vi "Min si Max Lab 2.vi"() -> ()   [LabVIEW 2023]
panel:
  out "Boolean":bool
  in  "Limitare":bool
  in  "MAX":dbl(slide) scale=0.0..10.0
  in  "MIN":dbl(slide) scale=0.0..10.0
  out "Tank":dbl(slide) scale=0.0..10.0
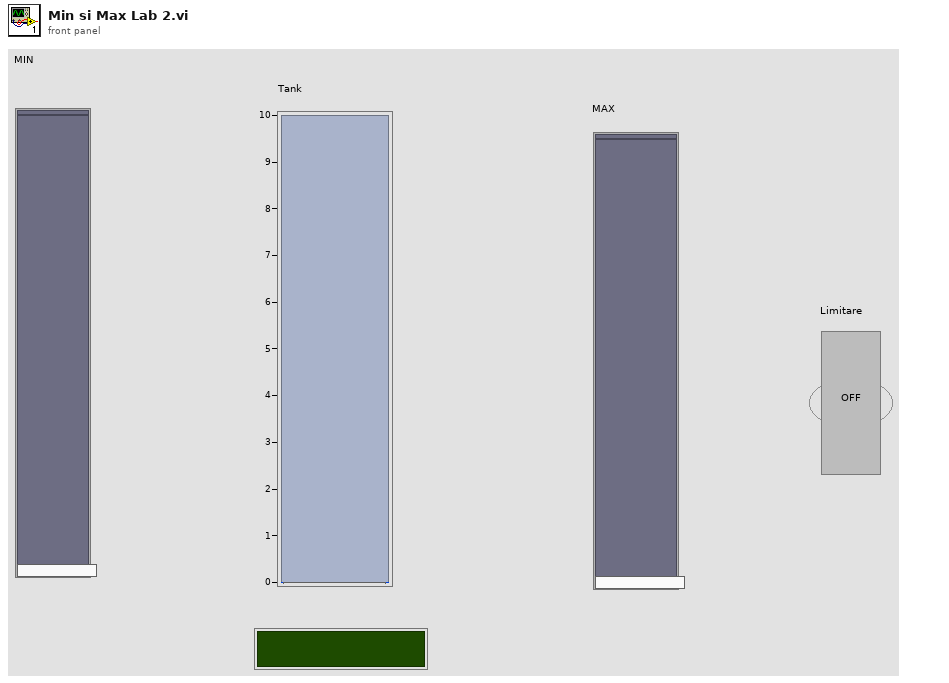
[diagram p1: front panel]
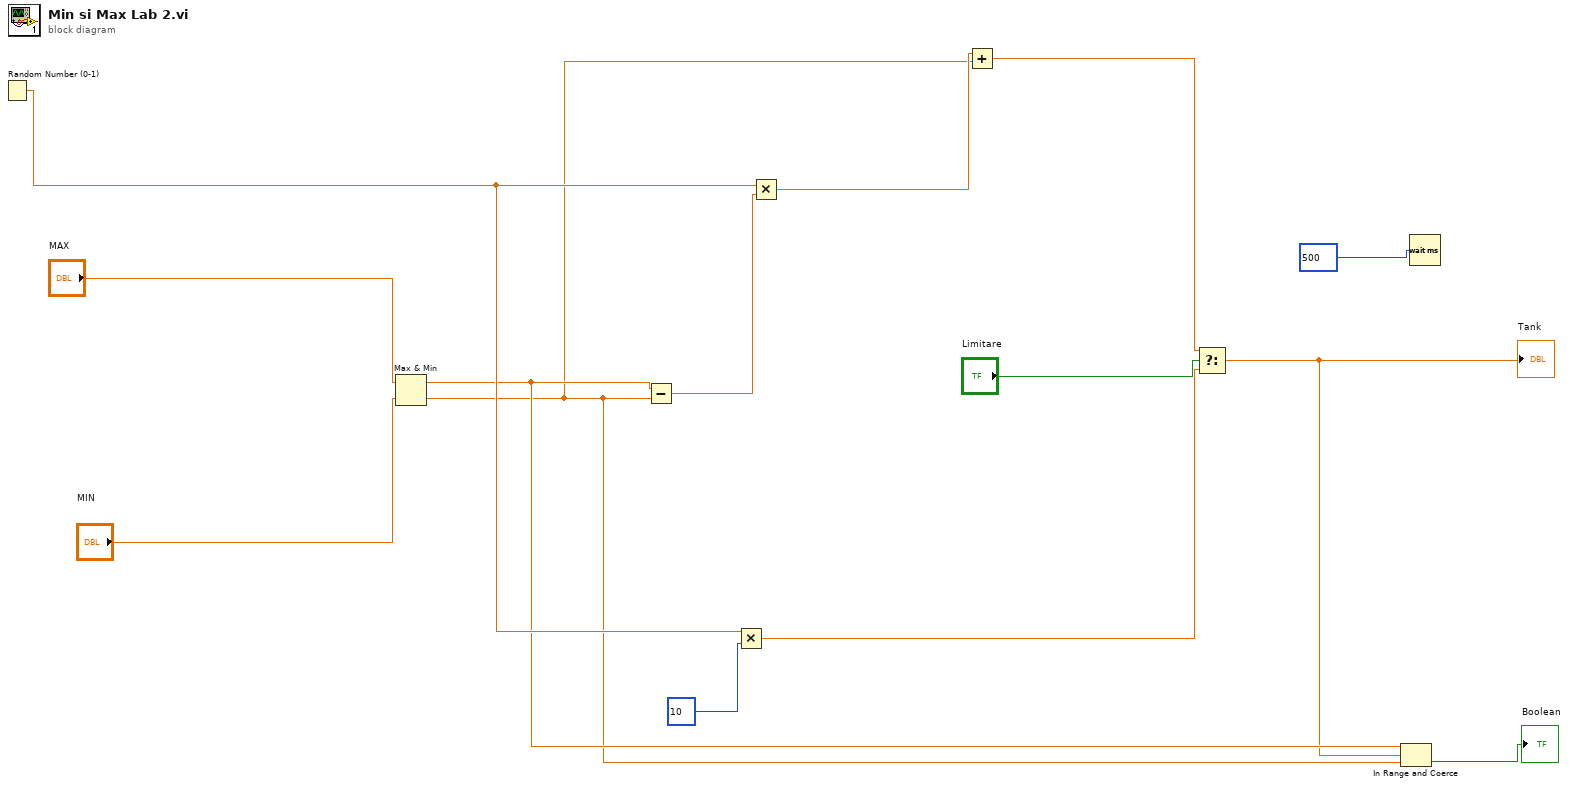
[diagram p0: block diagram]
diagram:
  n1 = Random Number (0-1)() -> (number: 0 to 1=w10:dbl)
  n2 = Max & Min(x="MAX", y="MIN") -> (max(x,y)=w5:dbl, min(x,y)=w3:dbl)
  n3 = Subtract(x=w5, y=w3) -> (x-y=w12:dbl)
  n4 = Multiply(x=w10, y=10) -> (x*y=w6:dbl)
  n5 = Multiply(x=w10, y=w12) -> (x*y=w11:dbl)
  n6 = Add(x=w11, y=w3) -> (x+y=w8:dbl)
  n7 = Select(t=w8, s="Limitare", f=w6) -> (s? t:f=w4:dbl)
  "Tank" <- w4
  n8 = In Range and Coerce(upper limit=w5, x=w4, lower limit=w3) -> (In Range?=→"Boolean":bool)  [unwired: 1 out]
  n9 = Wait (ms)(milliseconds to wait=500) -> ()  [unwired: 1 out]
